vi "Read Digital Input Module.vi"   [LabVIEW 2020, in "Scan Engine Scripting.lvlib"]
doc: "Returns the channel settings of a digital input module that can be edited and then used to create a new module instance to set into a slot."
uses:
  Scan Engine Scripting.lvlib
  Modules/NI 9422/NI 9422.lvclass
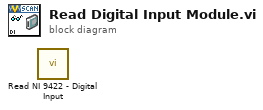
[diagram p0: block diagram]
diagram:
  n1 = call "Read NI 9422 - Digital Input.vi"() -> ()  [unwired: 9 in, 3 out]
